vi "数字到ID号---.vi"(8 "数值?":bool, 9 "字符串":string, 10 "数值":i32, 11 "个数":i32=4) -> (0 "连接的字符串":string, 1 "数组":string[](array[string]), 2 "十进制整型字符串":string, 3 "子字符串":string, 4 "16进制数据":string)   [LabVIEW 2014]
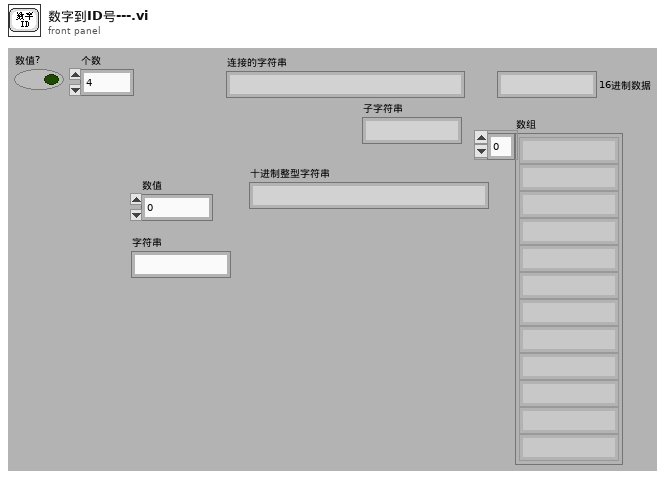
[diagram p1: front panel]
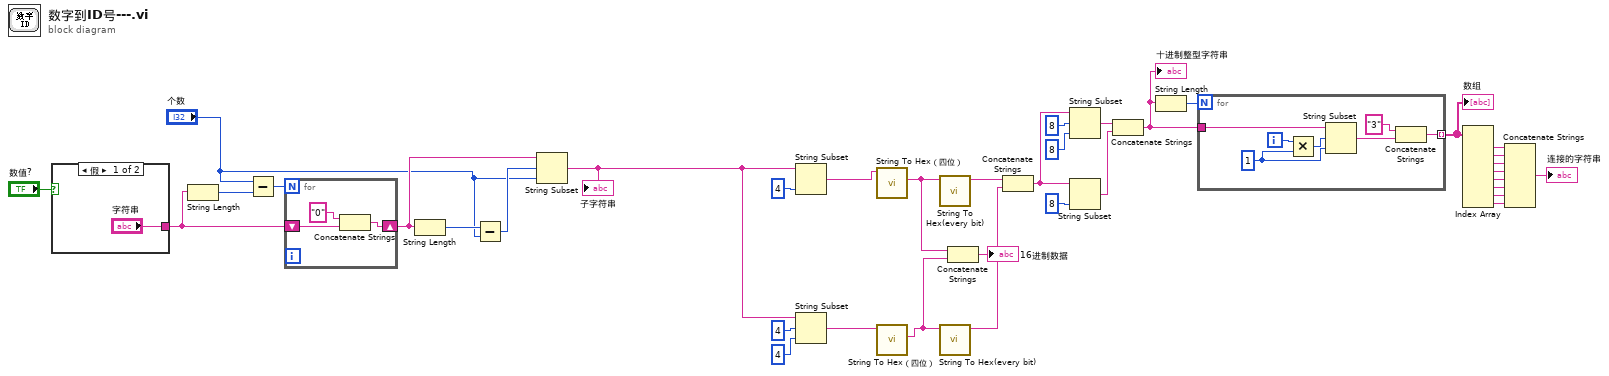
[diagram p0: block diagram]
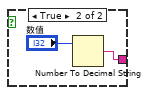
[diagram p2: hidden frame]
diagram:
  n1 = case shown="假" "数值?" {
    tunnel: ["字符串" w40] -> w35
    frame False {
    }
    frame True {
      n2 = Number To Decimal String(number="数值") -> (decimal integer string=w40:string)  [unwired: 1 in]
    }
  }
  n3 = String Length(string=w35) -> (length=w37:i32)
  n4 = Subtract(x="个数", y=w37) -> (x-y=w36:i32)
  n5 = for {
    N: w36 -> [_]
    shift-right: [w43] -> w34
    shift-left: w35 -> [w42]
    n6 = Concatenate Strings("0" ("字符串"), w42) -> (w43:string)
  }
  n7 = String Length(string=w34) -> (length=w33:i32)
  n8 = Subtract(x=w33, y="个数") -> (x-y=w32:i32)
  n9 = String Subset(string=w34, offset (0)=w32, length (rest)="个数") -> (substring=w11:string)
  "子字符串" <- w11
  n10 = String Subset(string=w11, length (rest)=4 ("长度（剩余）")) -> (substring=w9:string)  [unwired: 1 in]
  n11 = String Subset(string=w11, offset (0)=4 ("长度（剩余）"), length (rest)=4 ("长度（剩余）")) -> (substring=w10:string)
  n12 = call "String To Hex（四位）.vi"("String"=w9) -> ("低位"=w3:string)  [unwired: 6 in, 4 out]
  n13 = call "String To Hex（四位）.vi"("String"=w10) -> ("低位"=w2:string)  [unwired: 6 in, 4 out]
  n14 = call "String To Hex(every bit).vi"("字符串"=w3) -> ("十六进制整型字符串"=w6:string)  [unwired: 10 in]
  n15 = call "String To Hex(every bit).vi"("字符串"=w2) -> ("十六进制整型字符串"=w8:string)  [unwired: 10 in]
  n16 = Concatenate Strings(w3, w2) -> (→"16进制数据":string)
  n17 = Concatenate Strings(w6, w8) -> (w7:string)
  n18 = String Subset(string=w7, offset (0)=8 ("长度（剩余）"), length (rest)=8 ("长度（剩余）")) -> (substring=w17:string)
  n19 = String Subset(string=w7, length (rest)=8 ("长度（剩余）")) -> (substring=w16:string)  [unwired: 1 in]
  n20 = Concatenate Strings(w17, w16) -> (w15:string)
  "十进制整型字符串" <- w15
  n21 = String Length(string=w15) -> (length=w31:i32)
  n22 = for {
    N: w31 -> [_]
    tunnel: w15 -> [w50]
    tunnel: [w45] -> w30 mode=indexing
    i -> [w48]
    w47 = 1 ("y")
    n23 = Multiply(x=w48, y=w47) -> (x*y=w49:i32)
    n24 = String Subset(string=w50, offset (0)=w49, length (rest)=w47) -> (substring=w46:string)
    n25 = Concatenate Strings("3" ("字符串"), w46) -> (w45:string)
  }
  "数组" <- w30
  n26 = Index Array(array=w30) -> (element #1=w28:string, element #2=w29:string, element #3=w27:string, element #4=w26:string, element #5=w25:string, element #6=w24:string, element #7=w23:string, element #8=w22:string)  [unwired: 8 in]
  n27 = Concatenate Strings(w28, w29, w27, w26, w25, w24, w23, w22) -> (→"连接的字符串":string)
